vi "SetImageContrast.vi"(0 "CameraController in":refnum<class "CameraController.lvclass">, 5 "Image In":T1, 7 "Max":dbl(slide) scale=0.0..5000.0, 9 "Min":dbl(slide) scale=0.0..5000.0, 11 "error in (no error)":errorcluster) -> (4 "CameraController out":refnum<class "CameraController.lvclass">, 6 "Image Dst Out":T1, 15 "error out":errorcluster)   [LabVIEW 2020, in "CameraController.lvlib" / "CameraController.lvclass"]
uses:
  CameraController.lvclass
  <vilib>/vision/Image Controls.llb/IMAQ Image.ctl
  <vilib>/vision/NI_Vision_Development_Module.lvlib
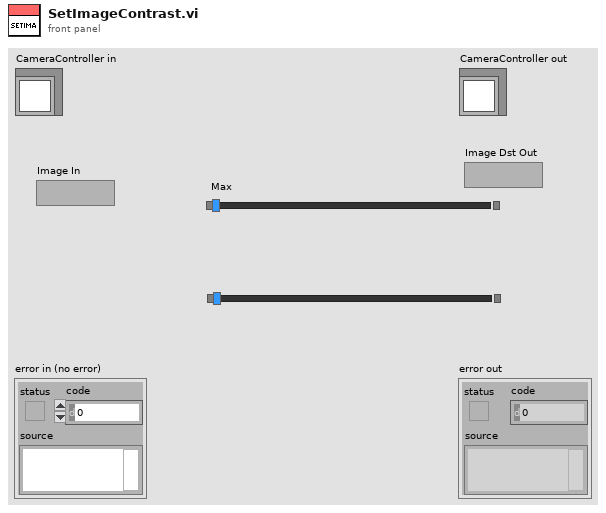
[diagram p1: front panel]
types:
  T1 = typedef "IMAQ Image.ctl" = refnum<image>
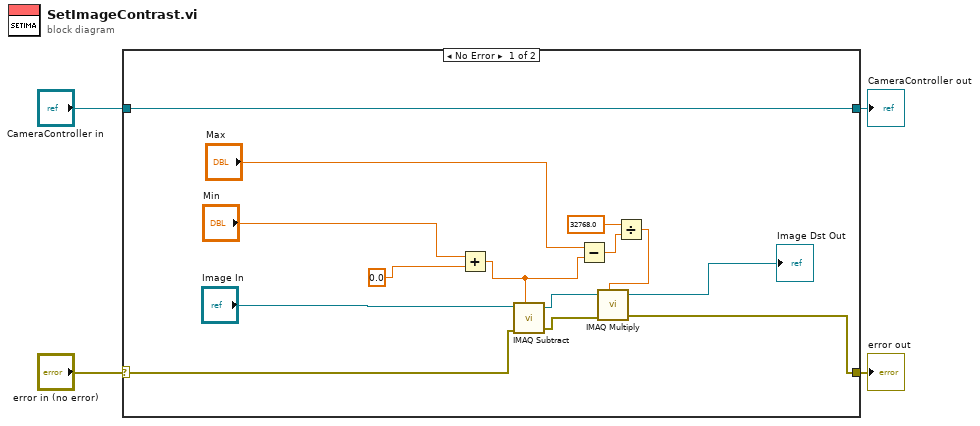
[diagram p0: block diagram]
diagram:
  n1 = case shown="No Error" "error in (no error)" {
    selector: "error in (no error)" -> [w7 w20]
    tunnel: [w5 w20] -> w3
    tunnel: [w18 w19] -> w1
    tunnel: "CameraController in" -> [w18 w19]
    frame No Error {
      n2 = Add(x="Min", y=0.0) -> (x+y=w16:dbl)
      n3 = call "IMAQ Subtract"("Image Src A"="Image In", "Constant"=w16, "error in (no error)"=w7) -> ("Image Dst Out"=w14:T1, "error out"=w6:errorcluster)  [unwired: 4 in]
      n4 = Subtract(x="Max", y=w16) -> (x-y=w12:dbl)
      n5 = Divide(x=32768.0, y=w12) -> (x/y=w13:dbl)
      n6 = call "IMAQ Multiply"("Image Src A"=w14, "Constant"=w13, "error in (no error)"=w6) -> ("Image Dst Out"=→"Image Dst Out":T1, "error out"=w5:errorcluster)  [unwired: 4 in]
    }
    frame Error {
    }
  }
  "error out" <- w3
  "CameraController out" <- w1
